vi "broadcast_common_trigger.vi"(8 "error in (no error)":errorcluster, 10 "trigger":T1, 11 "GenericToplevelComponent in":refnum<class "GenericToplevelComponent.lvclass">) -> (0 "error out":errorcluster, 3 "GenericToplevelComponent out":refnum<class "GenericToplevelComponent.lvclass">)   [LabVIEW 2010, in "GenericToplevelComponent.lvclass"]
uses:
  GenericToplevelComponent.lvclass
  common_trigger_enum.ctl
  components/DAQ/GenericDAQ/GenericDAQ/GenericDAQ.lvclass
  components/ExperimentController/GenericExperimentController/GenericExperimentController/GenericExperimentController.lvclass
  components/ImageAssembler/GenericImageAssembler/GenericImageAssembler/GenericImageAssembler.lvclass
  components/Instrument/GenericInstrument/GenericInstrument/GenericInstrument.lvclass
  components/ScanHead/GenericScanHead/GenericScanHead/GenericScanHead.lvclass
  components/Analyser/GenericAnalyser/GenericAnalyser/GenericAnalyser.lvclass
  components/DataCollection/GenericDataCollection/GenericDataCollection/GenericDataCollection.lvclass
  components/Display/GenericDisplay/GenericDisplay/GenericDisplay.lvclass
  components/Stage/GenericStage/GenericStage/GenericStage.lvclass
  components/Stimulator/GenericStimulator/GenericStimulator/GenericStimulator.lvclass
  components/ImagingMode/GenericImagingMode/GenericImagingMode/GenericImagingMode.lvclass
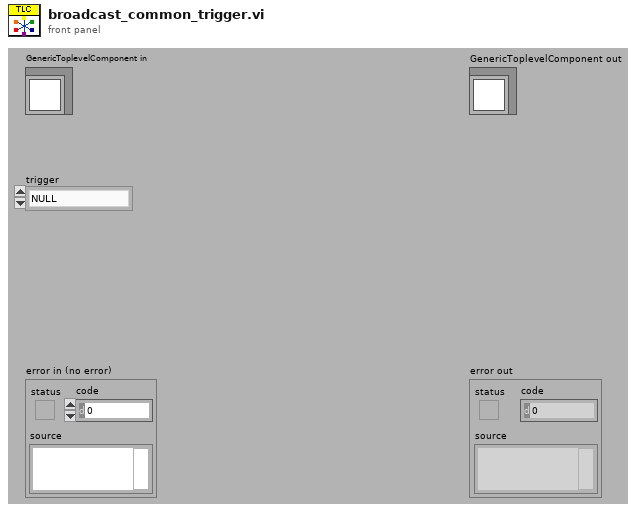
[diagram p1: front panel]
types:
  T1 = typedef "GenericToplevelComponent.lvclass/common_trigger_enum.ctl" = enum16{"NULL", "initialise", "terminate", "fetch command", "fetch data", "fetch image", "register as listener"}
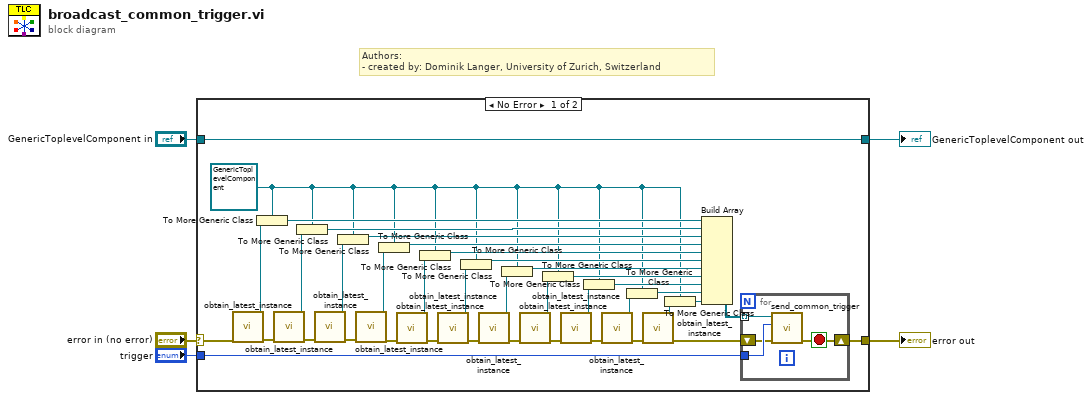
[diagram p0: block diagram]
diagram:
  # "Authors: \n- created by: Dominik Langer, University of Zurich, Switzerland"
  n1 = case shown="No Error" "error in (no error)" {
    selector: "error in (no error)" -> [w33 w50]
    tunnel: [w30 w50] -> w4
    tunnel: [w44 w49] -> w2
    tunnel: "GenericToplevelComponent in" -> [w44 w49]
    tunnel: "trigger" -> [w32 _]
    frame No Error {
      w7 = refnum<class "GenericToplevelComponent.lvclass"> refnum ("GenericToplevelComponent.lvclass")
      n2 = call "obtain_latest_instance.vi"("error in (no error)"=w33) -> ("error out"=w42:errorcluster, "GenericExperimentController out"=w29:refnum<class "GenericExperimentController.lvclass">)  [unwired: 9 in]
      n3 = To More Generic Class(target class=w7, reference=w29) -> (generic class reference=w25:refnum<class "GenericToplevelComponent.lvclass">)
      n4 = call "obtain_latest_instance.vi"("error in (no error)"=w42) -> ("error out"=w41:errorcluster, "GenericScanHead out"=w28:refnum<class "GenericScanHead.lvclass">)  [unwired: 9 in]
      n5 = To More Generic Class(target class=w7, reference=w28) -> (generic class reference=w24:refnum<class "GenericToplevelComponent.lvclass">)
      n6 = call "obtain_latest_instance.vi"("error in (no error)"=w41) -> ("error out"=w43:errorcluster, "GenericDAQ out"=w27:refnum<class "GenericDAQ.lvclass">)  [unwired: 9 in]
      n7 = To More Generic Class(target class=w7, reference=w27) -> (generic class reference=w23:refnum<class "GenericToplevelComponent.lvclass">)
      n8 = call "obtain_latest_instance.vi"("error in (no error)"=w43) -> ("error out"=w40:errorcluster, "GenericImageAssembler out"=w26:refnum<class "GenericImageAssembler.lvclass">)  [unwired: 9 in]
      n9 = To More Generic Class(target class=w7, reference=w26) -> (generic class reference=w22:refnum<class "GenericToplevelComponent.lvclass">)
      n10 = call "obtain_latest_instance.vi"("error in (no error)"=w40) -> ("error out"=w39:errorcluster, "GenericDisplay out"=w19:refnum<class "GenericDisplay.lvclass">)  [unwired: 9 in]
      n11 = To More Generic Class(target class=w7, reference=w19) -> (generic class reference=w21:refnum<class "GenericToplevelComponent.lvclass">)
      n12 = call "obtain_latest_instance.vi"("error in (no error)"=w39) -> ("error out"=w38:errorcluster, "GenericDataCollection out"=w18:refnum<class "GenericDataCollection.lvclass">)  [unwired: 9 in]
      n13 = To More Generic Class(target class=w7, reference=w18) -> (generic class reference=w20:refnum<class "GenericToplevelComponent.lvclass">)
      n14 = call "obtain_latest_instance.vi"("error in (no error)"=w38) -> ("error out"=w37:errorcluster, "GeneralAnalyser out"=w17:refnum<class "GenericAnalyser.lvclass">)  [unwired: 9 in]
      n15 = To More Generic Class(target class=w7, reference=w17) -> (generic class reference=w16:refnum<class "GenericToplevelComponent.lvclass">)
      n16 = call "obtain_latest_instance.vi"("error in (no error)"=w37) -> ("error out"=w36:errorcluster, "GenericScanMode out"=w15:refnum<class "GenericImagingMode.lvclass">)  [unwired: 9 in]
      n17 = To More Generic Class(target class=w7, reference=w15) -> (generic class reference=w13:refnum<class "GenericToplevelComponent.lvclass">)
      n18 = call "obtain_latest_instance.vi"("error in (no error)"=w36) -> ("error out"=w35:errorcluster, "GenericStimulator out"=w14:refnum<class "GenericStimulator.lvclass">)  [unwired: 9 in]
      n19 = To More Generic Class(target class=w7, reference=w14) -> (generic class reference=w12:refnum<class "GenericToplevelComponent.lvclass">)
      n20 = call "obtain_latest_instance.vi"("error in (no error)"=w35) -> ("error out"=w34:errorcluster, "microscope"=w11:refnum<class "GenericInstrument.lvclass">)  [unwired: 9 in]
      n21 = To More Generic Class(target class=w7, reference=w11) -> (generic class reference=w10:refnum<class "GenericToplevelComponent.lvclass">)
      n22 = call "obtain_latest_instance.vi"("error in (no error)"=w34) -> ("error out"=w31:errorcluster, "GenericStage out"=w9:refnum<class "GenericStage.lvclass">)  [unwired: 9 in]
      n23 = To More Generic Class(target class=w7, reference=w9) -> (generic class reference=w8:refnum<class "GenericToplevelComponent.lvclass">)
      n24 = Build Array(w25, w24, w23, w22, w21, w20, w16, w13, w12, w10, w8) -> (w6:refnum<class "GenericToplevelComponent.lvclass">[])
      n25 = for {
        tunnel: w32 -> [w48]
        shift-right: [w45] -> w30
        shift-left: w31 -> [w47]
        tunnel: w6 -> [w46] mode=indexing
        stop <- w45 stop-if-true
        n26 = call-dynamic "send_common_trigger.vi"("error in (no error)"=w47, "trigger"=w48, "GenericToplevelComponent in"=w46) -> ("error out"=w45:errorcluster)  [unwired: 7 in, 1 out]
      }
    }
    frame Error {
    }
  }
  "error out" <- w4
  "GenericToplevelComponent out" <- w2
